vi "SMS Candidate Selection - Pull Sub Regions.vi"(0 "Image Ref":T1, 7 "ROI Coordinates":i32[][](array[numeric]), 11 "Error":errorcluster) -> (4 "Image Ref (Dup)":T1, 8 "ROIs":u16[][][](array[numeric]), 15 "Error Out":errorcluster)   [LabVIEW 2016]
uses:
  <vilib>/vision/Image Controls.llb/IMAQ Image.ctl
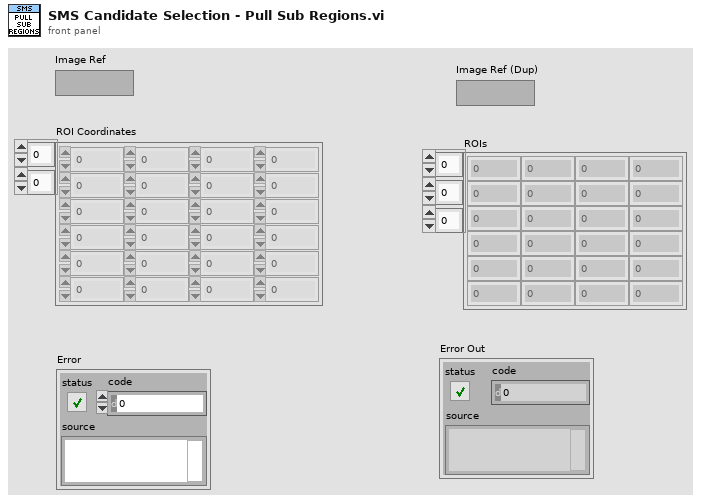
[diagram p1: front panel]
types:
  T1 = typedef "IMAQ Image.ctl" = refnum<image>
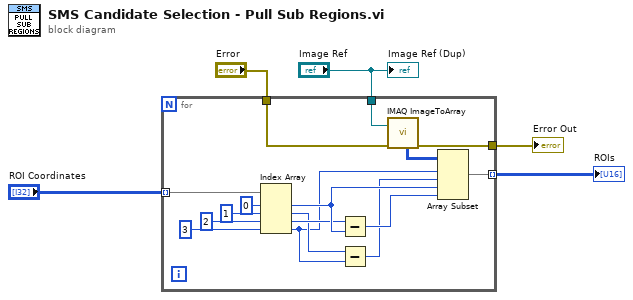
[diagram p0: block diagram]
diagram:
  n1 = for {
    tunnel: "Image Ref" -> [w17]
    tunnel: "ROI Coordinates" -> [w16] mode=indexing
    tunnel: [w8] -> w1 mode=indexing
    tunnel: "Error" -> [w7]
    tunnel: [w6] -> w2
    n2 = Index Array(array=w16, index #1=0 ("index"), index #2=1 ("index"), index #3=2 ("index"), index #4=3 ("index")) -> (element #1=w14:i32, element #2=w11:i32, element #3=w13:i32, element #4=w10:i32)
    n3 = Subtract(x=w13, y=w14) -> (x-y=w12:i32)
    n4 = Subtract(x=w11, y=w10) -> (x-y=w9:i32)
    n5 = call "IMAQ ImageToArray"("error in (no error)"=w7, "Image"=w17) -> ("Image Pixels (U16)"=w15:u16[][], "error out"=w6:errorcluster)  [unwired: 2 in, 3 out]
    n6 = Array Subset(array=w15, index (row)=w10, length (row)=w9, index (col)=w14, length (col)=w12) -> (w8:u16[][])
  }
  "Error Out" <- w2
  "ROIs" <- w1
  "Image Ref (Dup)" <- "Image Ref"
